vi "Command Settings.vi"() -> (5 "Command Settings":T1[](array[typedef])=[{"Enum"=enum."Start", "U8"=0, " Payload"=TRUE}, {"Enum"=enum."StartFTE", "U8"=0, " Payload"=FALSE}, {"Enum"=enum."Pause", "U8"=0, " Payload"=TRUE}, {"Enum"=enum."Stop", "U8"=0, " Payload"=TRUE}, {"Enum"=enum."Restart", "U8"=0, " Payload"=TRUE}, {"Enum"=enum."RestartFTE", "U8"=0, " Payload"=FALSE}, {"Enum"=enum."RefreshStats", "U8"=0, " Payload"=TRUE}, {"Enum"=enum."UpdateConfig", "U8"=0, " Payload"=FALSE}, {"Enum"=enum."Start", "U8"=0, " Payload"=FALSE}, {"Enum"=enum."UpdateConfig", "U8"=0, " Payload"=FALSE}])   [LabVIEW 2021, in "CIFCoreOOB_Rx.lvclass"]
uses:
  CIFCoreOOB_Rx.lvclass
  Typedef/Command Setting Control.ctl
  Typedef/OOB Core Commands.ctl
  CIFCoreOOB_Rx.lvclass/CIFCoreOOB_Rx.ctl
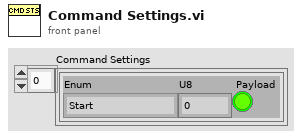
[diagram p1: front panel]
types:
  T1 = typedef "CIFCoreOOB_Rx.lvclass/Command Setting Control.ctl" = cluster{"Enum":T2, "U8":u8, " Payload":bool}
  T2 = typedef "CIFCoreOOB_Rx.lvclass/OOB Core Commands.ctl" = enum8{"Start", "StartFTE", "Pause", "Stop", "Restart", "RestartFTE", "RefreshStats", "UpdateConfig"}
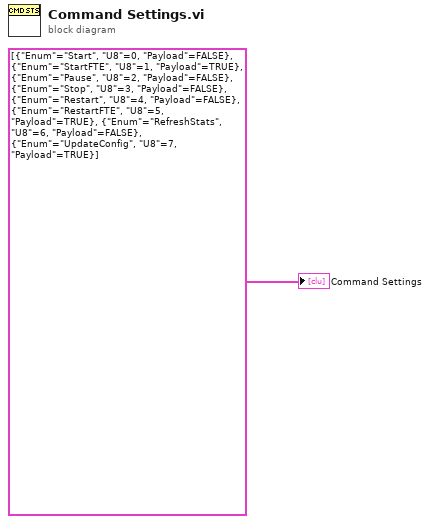
[diagram p0: block diagram]
diagram:
  "Command Settings" <- cluster{"Enum":T2, "U8":u8, "Payload":bool}[] [{"Enum"=enum."Start", "U8"=0, "Payload"=FALSE}, {"Enum"=enum."StartFTE", "U8"=1, "Payload"=TRUE}, {"Enum"=enum."Pause", "U8"=2, "Payload"=FALSE}, {"Enum"=enum."Stop", "U8"=3, "Payload"=FALSE}, {"Enum"=enum."Restart", "U8"=4, "Payload"=FALSE}, {"Enum"=enum."RestartFTE", "U8"=5, "Payload"=TRUE}, {"Enum"=enum."RefreshStats", "U8"=6, "Payload"=FALSE}, {"Enum"=enum."UpdateConfig", "U8"=7, "Payload"=TRUE}]
